vi "Initialize Parameter to Hardware Map from Experiment Cluster.vi"(8 "error in (no error)":errorcluster, 11 "Reaction Rover Data in":T1={"Main VI Queue"=refnum, "Process Queue References"=[], "Message Queue"=refnum, "Visible Hardware VI"="", "Current Message"={"Source"="", "Destination"="", "Time Stamp"=timestamp(0 s since 1904-01-01), "Command"="", "Data"=variant(string "")}, "Message History"=[], "Hardware"={"Process Cache"=refnum, "Plugins"=[{"Plugin Name"="ChromTech Pump Controller", "Controller Type"=enum."Invalid", "Control Panel Path"=path "", "Plugin Type"=enum."Optimizer"}, {"Plugin Name"="Pump Controller", "Controller Type"=enum."Invalid", "Control Panel Path"=path "", "Plugin Type"=enum."Optimizer"}, {"Plugin Name"="..\\Instrumentation\\ChromTech MX-Class\\Control Panel\\Main.vi", "Controller Type"=enum."Invalid", "Control Panel Path"=path "", "Plugin Type"=enum."Optimizer"}, {"Plugin Name"="", "Controller Type"=enum."Invalid", "Control Panel Path"=path "", "Plugin Type"=enum."Optimizer"}]}, "Optimizers"={"Process Cache"=refnum, "Plugins"=[{"Plugin Name"="Deep Reaction Optimizer", "Controller Type"=enum."Invalid", "Control Panel Path"=path "", "Plugin Type"=enum."Optimizer"}, {"Plugin Name"="..\\Optimizers\\Deep Reaction Optimizer\\Control Panel\\Main.vi", "Controller Type"=enum."Invalid", "Control Panel Path"=path "", "Plugin Type"=enum."Optimizer"}, {"Plugin Name"="..\\Optimizers\\Deep Reaction Optimizer\\Source - zmq\\start_inference.bat", "Controller Type"=enum."Invalid", "Control Panel Path"=path "", "Plugin Type"=enum."Optimizer"}], "First parameters?"=FALSE, "New Parameters"={"Time Stamp"=timestamp(0 s since 1904-01-01), "Names"=[], "Values"=[]}}, "Parameter to Hardware Map"=refnum, "Analyzers"={"Process Cache"=refnum, "Plugins"=[{"Plugin Name"="ChromTech Pump Controller", "Controller Type"=enum."Invalid", "Control Panel Path"=path "", "Plugin Type"=enum."Optimizer"}, {"Plugin Name"="Pump Controller", "Controller Type"=enum."Invalid", "Control Panel Path"=path "", "Plugin Type"=enum."Optimizer"}, {"Plugin Name"="..\\Instrumentation\\ChromTech MX-Class\\Control Panel\\Main.vi", "Controller Type"=enum."Invalid", "Control Panel Path"=path "", "Plugin Type"=enum."Optimizer"}, {"Plugin Name"="", "Controller Type"=enum."Invalid", "Control Panel Path"=path "", "Plugin Type"=enum."Optimizer"}]}, "Log Directory"=path "", "Auto Pass Parameters"=FALSE, "Experiment"={"Name"="", "File Path"=path "", "File Extension"="", "File Cluster"={"Hardware List"=[], "Optimizer List"=[], "Analyzer List"=[], "Parameter to Hardware Map"=[]}}}) -> (0 "error out":errorcluster, 3 "Reaction Rover Data out":T1={"Main VI Queue"=refnum, "Process Queue References"=[], "Message Queue"=refnum, "Visible Hardware VI"="", "Current Message"={"Source"="", "Destination"="", "Time Stamp"=timestamp(0 s since 1904-01-01), "Command"="", "Data"=variant(string "")}, "Message History"=[], "Hardware"={"Process Cache"=refnum, "Plugins"=[{"Plugin Name"="ChromTech Pump Controller", "Controller Type"=enum."Invalid", "Control Panel Path"=path "", "Plugin Type"=enum."Optimizer"}, {"Plugin Name"="Pump Controller", "Controller Type"=enum."Invalid", "Control Panel Path"=path "", "Plugin Type"=enum."Optimizer"}, {"Plugin Name"="..\\Instrumentation\\ChromTech MX-Class\\Control Panel\\Main.vi", "Controller Type"=enum."Invalid", "Control Panel Path"=path "", "Plugin Type"=enum."Optimizer"}, {"Plugin Name"="", "Controller Type"=enum."Invalid", "Control Panel Path"=path "", "Plugin Type"=enum."Optimizer"}]}, "Optimizers"={"Process Cache"=refnum, "Plugins"=[{"Plugin Name"="Deep Reaction Optimizer", "Controller Type"=enum."Invalid", "Control Panel Path"=path "", "Plugin Type"=enum."Optimizer"}, {"Plugin Name"="..\\Optimizers\\Deep Reaction Optimizer\\Control Panel\\Main.vi", "Controller Type"=enum."Invalid", "Control Panel Path"=path "", "Plugin Type"=enum."Optimizer"}, {"Plugin Name"="..\\Optimizers\\Deep Reaction Optimizer\\Source - zmq\\start_inference.bat", "Controller Type"=enum."Invalid", "Control Panel Path"=path "", "Plugin Type"=enum."Optimizer"}], "First parameters?"=FALSE, "New Parameters"={"Time Stamp"=timestamp(0 s since 1904-01-01), "Names"=[], "Values"=[]}}, "Parameter to Hardware Map"=refnum, "Analyzers"={"Process Cache"=refnum, "Plugins"=[{"Plugin Name"="ChromTech Pump Controller", "Controller Type"=enum."Invalid", "Control Panel Path"=path "", "Plugin Type"=enum."Optimizer"}, {"Plugin Name"="Pump Controller", "Controller Type"=enum."Invalid", "Control Panel Path"=path "", "Plugin Type"=enum."Optimizer"}, {"Plugin Name"="..\\Instrumentation\\ChromTech MX-Class\\Control Panel\\Main.vi", "Controller Type"=enum."Invalid", "Control Panel Path"=path "", "Plugin Type"=enum."Optimizer"}, {"Plugin Name"="", "Controller Type"=enum."Invalid", "Control Panel Path"=path "", "Plugin Type"=enum."Optimizer"}]}, "Log Directory"=path "", "Auto Pass Parameters"=FALSE, "Experiment"={"Name"="", "File Path"=path "", "File Extension"="", "File Cluster"={"Hardware List"=[], "Optimizer List"=[], "Analyzer List"=[], "Parameter to Hardware Map"=[]}}})   [LabVIEW 2020]
uses:
  Type Definitions/Data.ctl
  Plugin Servers/Controller Array/Controller Array.lvclass
  Plugin Servers/Parameter to Hardware Map/Parameter to Hardware Map.lvclass
  <userlib>/RxnRover/DynamicReentrant/src/Type Defs/Message.ctl
  Plugin Manager/Plugin Details.ctl
  Plugin Servers/Controller/Controller Type.ctl
  Plugin Manager/Plugin Types.ctl
  Experiment/Experiment File/Experiment File Cluster.ctl
  Plugin Servers/Controller/Minimal Controller Cluster.ctl
  Plugin Servers/Parameter to Hardware Map/Minimal Map.ctl
  Plugin Servers/Parameter to Hardware Map/Minimal Pair Cluster.ctl
  <userlib>/RxnRover/DynamicReentrant/Dynamic Reentrant.lvlib
  Plugin Servers/Controller/Generic Plugin.lvclass
  Experiment/Experiment File/Experiment File.lvlib
  Plugin Manager/Plugin Manager.lvlib
panel:
  # "Note: Rxn Rover data control and indicator are hidden!"
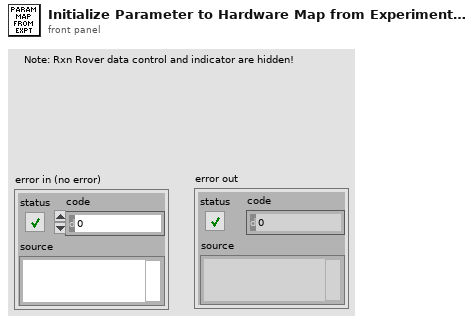
[diagram p1: front panel]
types:
  T1 = typedef "Data.ctl" = cluster{"Main VI Queue":refnum<queue>, "Process Queue References":refnum<queue>[], "Message Queue":refnum<queue>, "Visible Hardware VI":string, "Current Message":T2, "Message History":string[][], "Hardware":cluster{"Process Cache":refnum<class "Controller Array.lvclass">, "Plugins":T3[]}, "Optimizers":cluster{"Process Cache":refnum<class "Controller Array.lvclass">, "Plugins":T3[], "First parameters?":bool, "New Parameters":cluster{"Time Stamp":timestamp, "Names":string[], "Values":dbl[]}}, "Parameter to Hardware Map":refnum<class "Parameter to Hardware Map.lvclass">, "Analyzers":cluster{"Process Cache":refnum<class "Controller Array.lvclass">, "Plugins":T3[]}, "Log Directory":path, "Auto Pass Parameters":bool, "Experiment":cluster{"Name":string, "File Path":path, "File Extension":string, "File Cluster":T6}}
  T2 = typedef "Dynamic Reentrant.lvlib/Message.ctl" = cluster{"Source":string, "Destination":string, "Time Stamp":timestamp, "Command":string, "Data":variant}
  T3 = typedef "Plugin Manager.lvlib/Plugin Details.ctl" = cluster{"Plugin Name":string, "Controller Type":T4, "Control Panel Path":path, "Plugin Type":T5}
  T4 = typedef "Generic Plugin.lvclass/Controller Type.ctl" = enum16{"Invalid", "Temperature Controller", "Pump Controller", "Generic Optimizer", "LC Parser"}
  T5 = typedef "Plugin Manager.lvlib/Plugin Types.ctl" = enum16{"Invalid", "Optimizer", "Analyzer", "Hardware"}
  T6 = typedef "Experiment File.lvlib/Experiment File Cluster.ctl" = cluster{"Hardware List":T7[], "Optimizer List":T7[], "Analyzer List":T7[], "Parameter to Hardware Map":T8}
  T7 = typedef "Generic Plugin.lvclass/Minimal Controller Cluster.ctl" = cluster{"Name":string, "Controller Type":string, "Control Panel Path":string, "Resource":string}
  T8 = typedef "Parameter to Hardware Map.lvclass/Minimal Map.ctl" = T9[]
  T9 = typedef "Parameter to Hardware Map.lvclass/Minimal Pair Cluster.ctl" = cluster{"key":string, "values":T7[]}
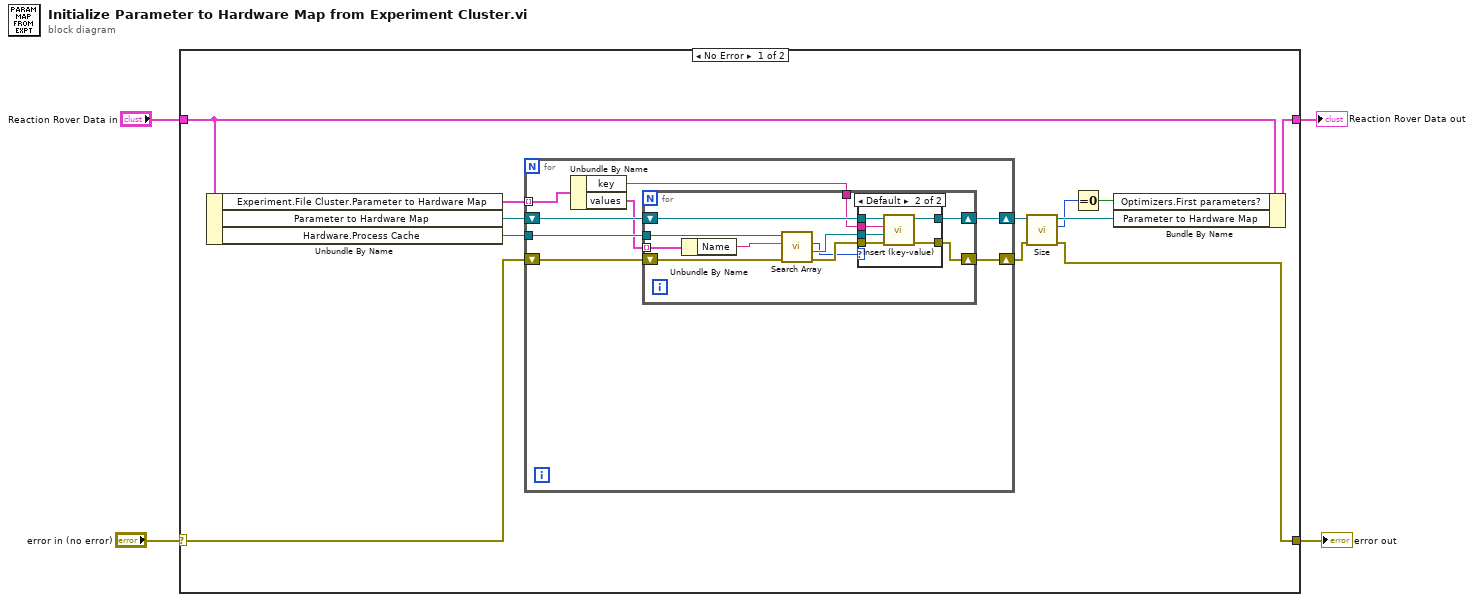
[diagram p0: block diagram]
diagram:
  n1 = case shown="No Error" "error in (no error)" {
    selector: "error in (no error)" -> [w12 w45]
    tunnel: [w5 w45] -> w3
    tunnel: [w11 w44] -> w1
    tunnel: "Reaction Rover Data in" -> [w16 w44]
    frame No Error {
      n2 = Unbundle By Name(w16) -> ("Experiment.File Cluster.Parameter to Hardware Map"=w15:T8, "Parameter to Hardware Map"=w14:refnum<class "Parameter to Hardware Map.lvclass">, "Hardware.Process Cache"=w13:refnum<class "Controller Array.lvclass">)
      n3 = for {
        tunnel: w15 -> [w23] mode=indexing
        tunnel: w13 -> [w21]
        shift-right: [w18] -> w6
        shift-left: w12 -> [w19]
        shift-right: [w17] -> w10
        shift-left: w14 -> [w24]
        n4 = Unbundle By Name(w23) -> ("key"=w22:string, "values"=w20:T7[])
        n5 = for {
          tunnel: w22 -> [w34]
          tunnel: w21 -> [w33]
          tunnel: w20 -> [w32] mode=indexing
          shift-right: [w26] -> w18
          shift-left: w19 -> [w31]
          shift-right: [w27] -> w17
          shift-left: w24 -> [w35]
          n6 = Unbundle By Name(w32) -> ("Name"=w25:string)
          n7 = call "Search Array.vi"("error in (no error)"=w31, "Search Value"=w25, "Controller Array in"=w33) -> ("error out"=w30:errorcluster, "Controller found"=w29:refnum<class "Generic Plugin.lvclass">, "Index of found"=w28:i32)  [unwired: 1 in, 1 out]
          n8 = case shown="Default" w28 {
            tunnel: w35 -> [w37 w43]
            tunnel: w34 -> [_ w42]
            tunnel: w30 -> [w36 w41]
            tunnel: w29 -> [_ w40]
            tunnel: [w37 w39] -> w27
            tunnel: [w36 w38] -> w26
            frame -1 {
            }
            frame Default {
              n9 = call "Insert (key-value).vi"("error in (no error)"=w41, "Value"=w40, "Key"=w42, "Parameter to Hardware Map in"=w43) -> ("error out"=w38:errorcluster, "Parameter to Hardware Map out"=w39:refnum<class "Parameter to Hardware Map.lvclass">)  [unwired: 6 in]
            }
          }
        }
      }
      n10 = call "Size.vi"("error in (no error)"=w6, "Parameter to Hardware Map in"=w10) -> ("error out"=w5:errorcluster, "Size"=w7:i32, "Parameter to Hardware Map out"=w9:refnum<class "Parameter to Hardware Map.lvclass">)  [unwired: 7 in]
      n11 = Equal To 0?(x=w7) -> (x = 0?=w8:bool)
      n12 = Bundle By Name(cluster=w16, "Optimizers.First parameters?"=w8, "Parameter to Hardware Map"=w9) -> (w11:T1)
    }
    frame Error {
    }
  }
  "Reaction Rover Data out" <- w1
  "error out" <- w3
